vi "Configure.vi"(8 "error in (no error)":errorcluster, 11 "Murmex in":refnum<class "ExampleClassB.lvclass">) -> (0 "error out":errorcluster, 2 "cancelled?":bool, 3 "Murmex out":refnum<class "ExampleClassB.lvclass">)   [LabVIEW 2012, in "ExampleClassB.lvclass"]
doc: "The configure method configures the details for the RabbitMQ connection. \n\nIn the derived class, make a call to the parent for setting these parameters."
uses:
  ExampleClassB.lvclass
  ExampleClassB.lvclass/ExampleClassB.ctl
  <vilib>/Distrio/Murmex/Murmex/Murmex.lvclass
panel:
  out "label":string
  in  "button:configureParent":bool
  in  "button:cancel":bool
  in  "button:ok":bool
  in  "Offset":dbl
  in  "Scaling factor":dbl
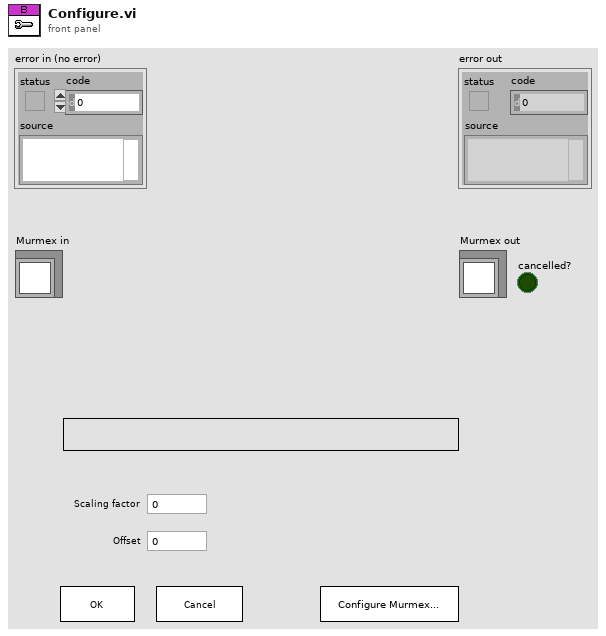
[diagram p1: front panel]
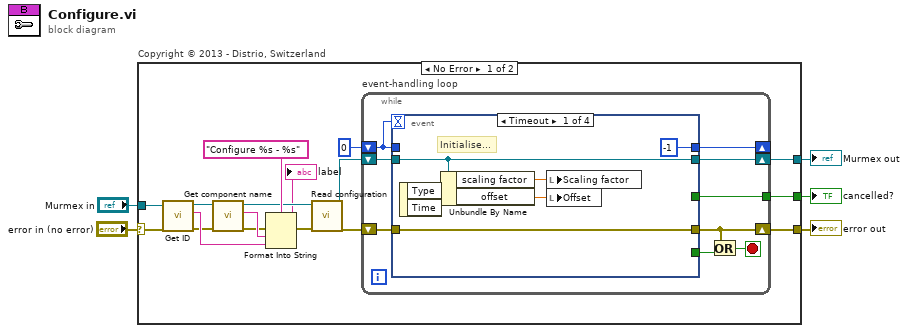
[diagram p0: block diagram]
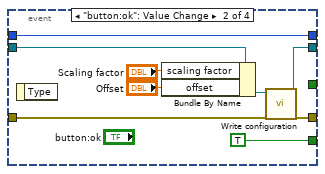
[diagram p2: hidden frame]
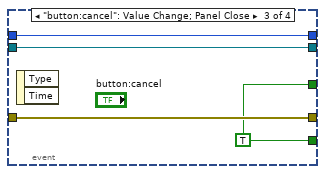
[diagram p3: hidden frame]
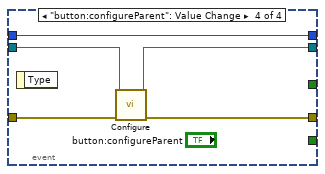
[diagram p4: hidden frame]
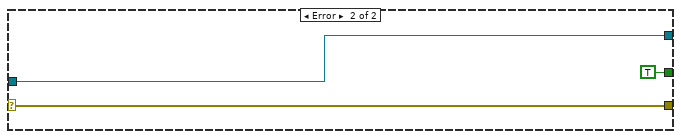
[diagram p5: hidden frame]
diagram:
  n1 = case "Copyright © 2013 - Distrio, Switzerland" shown="No Error" "error in (no error)" {
    selector: "error in (no error)" -> [w10 w57]
    tunnel: "Murmex in" -> [w8 w56]
    tunnel: [w22 w56] -> w3
    tunnel: [w21 w57] -> w2
    tunnel: [w6 TRUE] -> w1
    frame No Error {
      n2 = call <vilib>:"Get ID.vi"("error in (no error)"=w10, "Murmex in"=w8) -> ("error out"=w16:errorcluster, "component id"=w19:string, "Murmex out"=w17:refnum<class "ExampleClassB.lvclass">)  [unwired: 7 in]
      n3 = call <vilib>:"Get component name.vi"("error in (no error)"=w16, "Murmex in"=w17) -> ("error out"=w15:errorcluster, "component name"=w18:string, "Murmex out"=w12:refnum<class "ExampleClassB.lvclass">)  [unwired: 7 in]
      n4 = Format Into String(format string="Configure %s - %s" ("string"), error in=w15, w18, w19) -> (resulting string=→"label":string, error out=w14:errorcluster)  [unwired: 1 in]
      n5 = call <vilib>:"Read configuration.vi"("error in (no error)"=w14, "Murmex in"=w12) -> ("error out"=w9:errorcluster, "Murmex out"=w7:refnum<class "ExampleClassB.lvclass">)  [unwired: 7 in, 1 out]
      n6 = while "event-handling loop" {
        shift-right: [w27] -> w21
        shift-left: w9 -> [w31]
        shift-right: [w29] -> w22
        shift-left: w7 -> [w30]
        shift-right: [w24] -> _
        shift-left: 0 -> [w25]
        tunnel: [w23] -> w6
        stop <- w26 stop-if-true
        n7 = event shown="[0] Timeout" {
          selector: _ -> [_ _ _ _]
          dyn-events: _ -> [_ _ _ _]
          timeout: w25 -> [_ _ _ _]
          tunnel: w31 -> [w36 w40 w49 w51]
          tunnel: [w36 w39 w49 w50] -> w27
          tunnel: [w34 w37 w47 w52] -> w29
          tunnel: w30 -> [w34 w44 w47 w53]
          tunnel: [_ TRUE w46 _] -> w28
          tunnel: [-1 w41 w48 w54] -> w24
          tunnel: w25 -> [_ w41 w48 w54]
          tunnel: [_ _ w46 _] -> w23
          event Timeout {
            # "Initialise..."
            n8 = event-data() -> ()  [unwired: 1 in, 2 out]
            n9 = Unbundle By Name(w34) -> ("scaling factor"=w32:dbl, "offset"=w33:dbl)
            n10 = local write "Scaling factor"(w32) -> ()
            n11 = local write "Offset"(w33) -> ()
          }
          event "button:ok": Value Change {
            n12 = event-data() -> ()  [unwired: 1 in, 1 out]
            n13 = Bundle By Name(cluster=w44, "scaling factor"="Scaling factor", "offset"="Offset") -> (w38:refnum<class "ExampleClassB.lvclass">)
            n14 = call <vilib>:"Write configuration.vi"("error in (no error)"=w40, "Murmex in"=w38) -> ("error out"=w39:errorcluster, "Murmex out"=w37:refnum<class "ExampleClassB.lvclass">)  [unwired: 8 in]
          }
          event "button:cancel": Value Change; Panel Close {
            w46 = TRUE
            n15 = event-data() -> ()  [unwired: 1 in, 2 out]
          }
          event "button:configureParent": Value Change {
            n16 = event-data() -> ()  [unwired: 1 in, 1 out]
            n17 = call-parent "Configure.vi"("error in (no error)"=w51, "Murmex in"=w53) -> ("error out"=w50:errorcluster, "Murmex out"=w52:refnum<class "ExampleClassB.lvclass">)  [unwired: 7 in, 1 out]
          }
        }
        n18 = Or(x=w27, y=w28) -> (x .or. y?=w26:bool)
      }
    }
    frame Error {
    }
  }
  "error out" <- w2
  "Murmex out" <- w3
  "cancelled?" <- w1
